vi "SwerveCenterKinematics.vi"(9 "J2X":dbl(slide) scale=-1.0..1.0, 10 "J1Y":dbl(slide) scale=-1.0..1.0, 11 "J1X":dbl(slide) scale=1.0..-1.0) -> (0 "Velocity 3 (ul)":dbl, 1 "Velocity 2 (ul)":dbl, 2 "Velocity 1 (ul)":dbl, 3 "Velocity 0 (ul)":dbl format="%.2f", 4 "Angle 2 (deg)":dbl, 5 "Angle 1 (deg)":dbl, 6 "Angle 3 (deg)":dbl, 7 "Angle 0 (deg)":dbl)   [LabVIEW 2019]
doc: "Performs the kinematics for a rectangular four wheel swerve robot with a center of rotation at the geometric center of the robot. Swerve module #0 is located in the front right corner and the modules increment in the counter-clockwise direction."
panel:
  out "Velocity 0 (ul) New":dbl format="%.2f"
  out "Angle 0 (deg) New":dbl
  in  "Rotation Center Y (in)":dbl
  in  "Rotation Center X (in)":dbl
  in  "Robot Width (in)":dbl=25.0
  in  "Robot Length (in)":dbl=25.0
  # "I think the new value is correct and we are masking \nit by interverting the rotation joystick motors"
  # "Left Thumbstick"
  # "Right Thumbstick"
  # "*** weird b/c of inversion\nin DriveStateController.vi***"
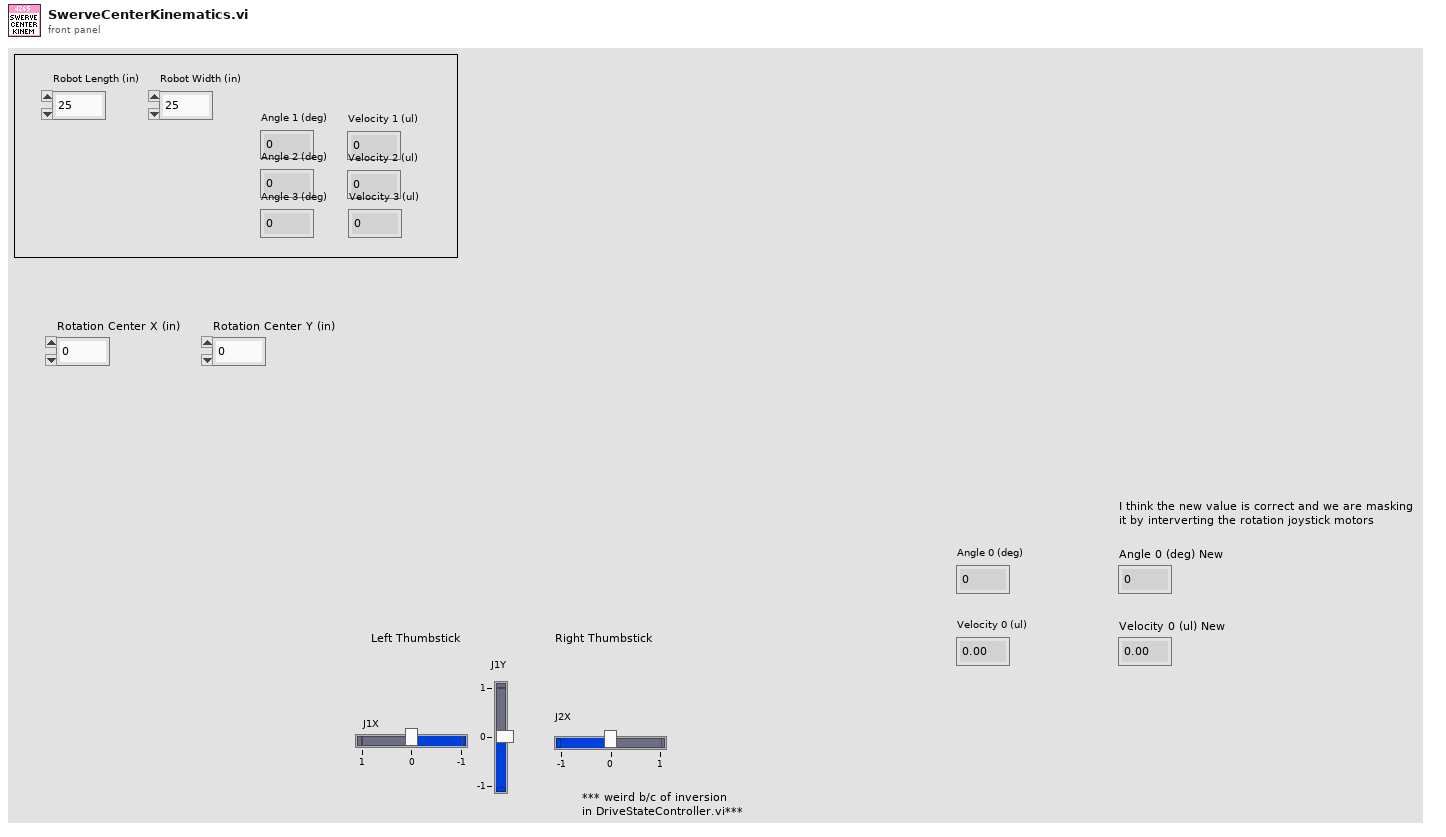
[diagram p1: front panel]
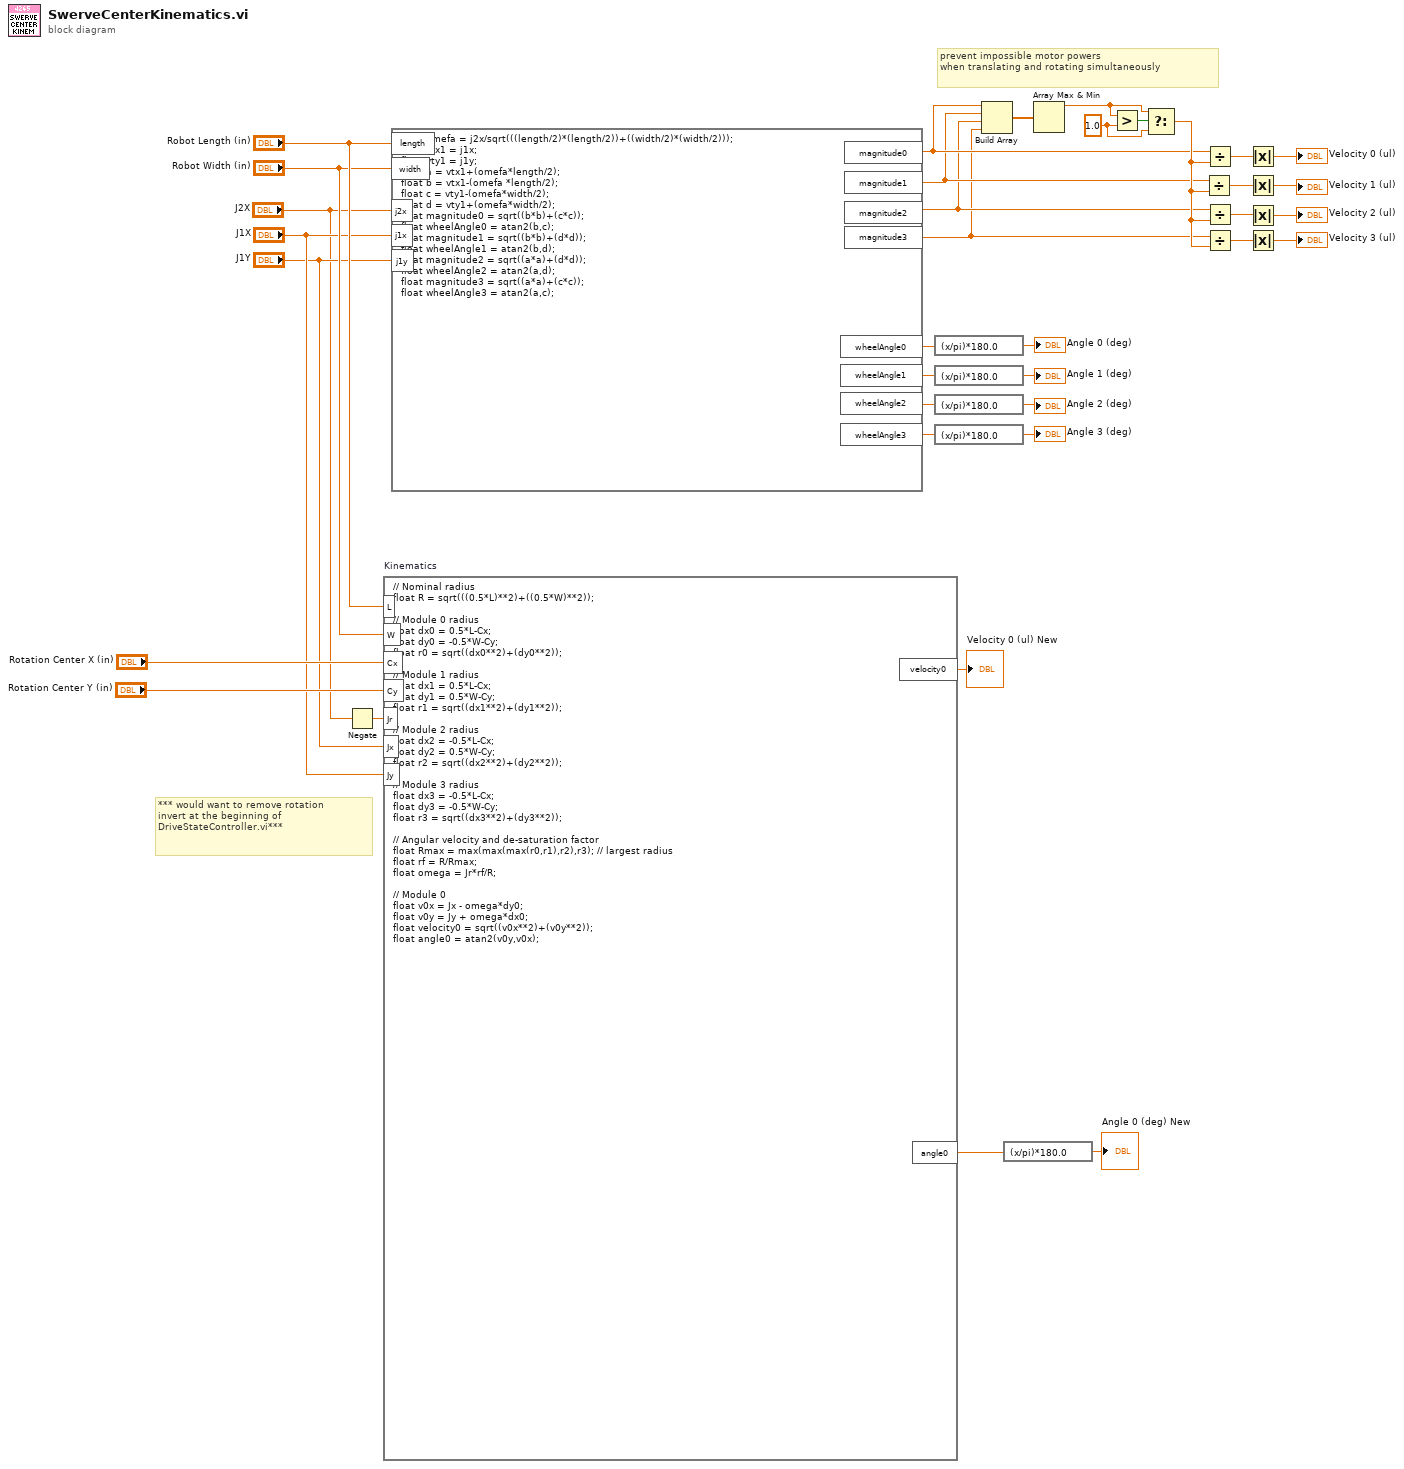
[diagram p0: block diagram]
diagram:
  w31 = 1.0 ("y")
  # "*** would want to remove rotation\ninvert at the beginning of\nDriveStateController.vi***"
  # "prevent impossible motor powers\nwhen translating and rotating simultaneously"
  n1 = Negate(x="J2X") -> (-x=w1:dbl)
  n2 = formula code="// Nominal radius\nfloat R = sqrt(((0.5*L)**2)+((0.5*W)**2));\n\n// Module 0 radius\nfloat dx0 = 0.5*L-Cx;\nfloat dy0 = -0.5*W-Cy;\nfloat r0 = sqrt((dx0**2)+(dy0**2));\n\n// Module 1 radius\nfloat dx1 = 0.5*L-Cx;\nfloat dy1 = 0.5*W-Cy;\nfloat r1 = sqrt((dx1**2)+(dy1**2));\n\n// Module 2 radius\nfloat dx2 = -0.5*L-Cx;\nfloat dy2 = 0.5*W-Cy;\nfloat r2 = sqrt((dx2**2)+(dy2**2));\n\n// Module 3 radius\nfloat dx3 = -0.5*L-Cx;\nfloat dy3 = -0.5*W-Cy;\nfloat r3 = sqrt((dx3**2)+(dy3**2));\n\n// Angular velocity and de-saturation factor\nfloat Rmax = max(max(max(r0,r1),r2),r3); // largest radius\nfloat rf = R/Rmax;\nfloat omega = Jr*rf/R;\n\n// Module 0\nfloat v0x = Jx - omega*dy0;\nfloat v0y = Jy + omega*dx0;\nfloat velocity0 = sqrt((v0x**2)+(v0y**2));\nfloat angle0 = atan2(v0y,v0x);" "Kinematics"("L"="Robot Length (in)", "W"="Robot Width (in)", "Cx"="Rotation Center X (in)", "Cy"="Rotation Center Y (in)", "Jr"=w1, "Jx"="J1Y", "Jy"="J1X") -> ("velocity0"=→"Velocity 0 (ul) New":dbl, "angle0"=w5:dbl)
  n3 = formula code="float omefa = j2x/sqrt(((length/2)*(length/2))+((width/2)*(width/2)));\nfloat vtx1 = j1x;\nfloat vty1 = j1y;\nfloat a = vtx1+(omefa*length/2);\nfloat b = vtx1-(omefa *length/2);\nfloat c = vty1-(omefa*width/2);\nfloat d = vty1+(omefa*width/2);\nfloat magnitude0 = sqrt((b*b)+(c*c));\nfloat wheelAngle0 = atan2(b,c);\nfloat magnitude1 = sqrt((b*b)+(d*d));\nfloat wheelAngle1 = atan2(b,d);\nfloat magnitude2 = sqrt((a*a)+(d*d));\nfloat wheelAngle2 = atan2(a,d);\nfloat magnitude3 = sqrt((a*a)+(c*c));\nfloat wheelAngle3 = atan2(a,c);"("length"="Robot Length (in)", "width"="Robot Width (in)", "j2x"="J2X", "j1y"="J1Y", "j1x"="J1X") -> ("wheelAngle0"=w17:dbl, "magnitude0"=w15:dbl, "magnitude1"=w14:dbl, "magnitude2"=w13:dbl, "magnitude3"=w12:dbl, "wheelAngle1"=w20:dbl, "wheelAngle2"=w22:dbl, "wheelAngle3"=w24:dbl)
  n4 = expression code="(x/pi)*180.0" ("radians to degrees")(w17) -> (→"Angle 0 (deg)":dbl)
  n5 = expression code="(x/pi)*180.0" ("radians to degrees")(w20) -> (→"Angle 1 (deg)":dbl)
  n6 = expression code="(x/pi)*180.0" ("radians to degrees")(w22) -> (→"Angle 2 (deg)":dbl)
  n7 = expression code="(x/pi)*180.0" ("radians to degrees")(w24) -> (→"Angle 3 (deg)":dbl)
  n8 = Build Array(w15, w14, w13, w12) -> (w16:dbl[])
  n9 = expression code="(x/pi)*180.0" ("radians to degrees")(w5) -> (→"Angle 0 (deg) New":dbl)
  n10 = Array Max & Min(array=w16) -> (max value=w30:dbl)  [unwired: 3 out]
  n11 = Greater?(x=w30, y=w31) -> (0:w32:bool)
  n12 = Select(t=w30, s=w32, f=w31) -> (s? t:f=w26:dbl)
  n13 = Divide(x=w14, y=w26) -> (x/y=w28:dbl)
  n14 = Divide(x=w15, y=w26) -> (x/y=w29:dbl)
  n15 = Divide(x=w13, y=w26) -> (x/y=w27:dbl)
  n16 = Divide(x=w12, y=w26) -> (x/y=w25:dbl)
  n17 = Absolute Value(x=w29) -> (abs(x)=→"Velocity 0 (ul)":dbl)
  n18 = Absolute Value(x=w28) -> (abs(x)=→"Velocity 1 (ul)":dbl)
  n19 = Absolute Value(x=w27) -> (abs(x)=→"Velocity 2 (ul)":dbl)
  n20 = Absolute Value(x=w25) -> (abs(x)=→"Velocity 3 (ul)":dbl)
